vi "setup_lc_zt.vi"(0 "shuoming":string, 1 "didian":string, 6 "jsren":string, 9 "yw":string, 10 "id":string, 11 "zc_luodi_num":string) -> (2 "error":errorcluster caption="error out 2")   [LabVIEW 2017, in "Lib_code.lvlib"]
uses:
  Lib_code.lvlib
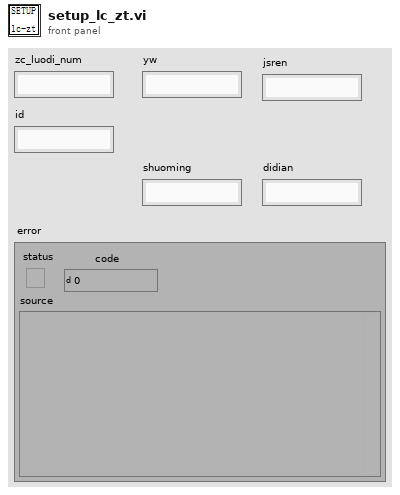
[diagram p1: front panel]
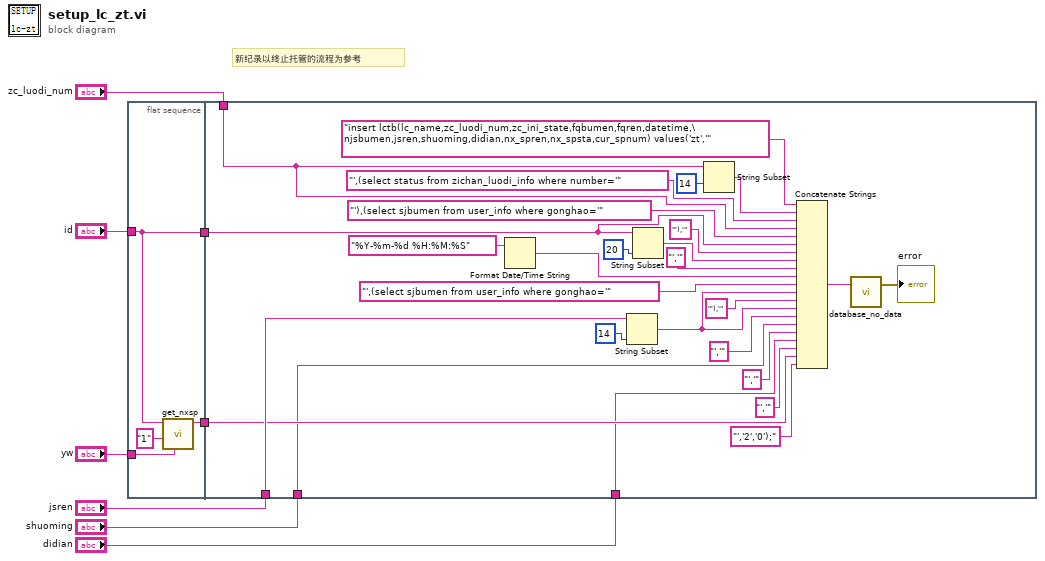
[diagram p0: block diagram]
diagram:
  # "新纪录以终止托管的流程为参考"
  n1 = flat-sequence {
    tunnel: "id" -> [w11]
    tunnel: [w11] -> w7
    tunnel: [w12] -> w6
    tunnel: "yw" -> [w10]
    tunnel: w7 -> [w20]
    tunnel: w6 -> [w28]
    tunnel: "zc_luodi_num" -> [w22]
    tunnel: "jsren" -> [w29]
    tunnel: "shuoming" -> [w16]
    tunnel: "didian" -> [w25]
    frame #0 {
      n2 = call "get_nxsp.vi"("yw"=w10, "Cur_state"="1", "fqren"=w11) -> ("sp_gonghao"=w12:string)  [unwired: 6 in, 2 out]
    }
    frame #1 {
      n3 = Format Date/Time String(time format string (%c)="%Y-%m-%d %H:%M:%S" ("时间格式字符串(%c)")) -> (date/time string=w15:string)  [unwired: 2 in]
      n4 = String Subset(string=w29, length (rest)=14 ("长度（剩余）")) -> (substring=w13:string)  [unwired: 1 in]
      n5 = String Subset(string=w20, length (rest)=20 ("长度（剩余）")) -> (substring=w32:string)  [unwired: 1 in]
      n6 = String Subset(string=w22, length (rest)=14 ("长度（剩余）")) -> (substring=w37:string)  [unwired: 1 in]
      n7 = Concatenate Strings("insert lctb(lc_name,zc_luodi_num,zc_ini_state,fqbumen,fqren,datetime,\njsbumen,jsren,shuoming,didian,nx_spren,nx_spsta,cur_spnum) values('zt','" ("格式字符串"), w37, "',(select status from zichan_luodi_info where number='" ("字符串"), w22, "'),(select sjbumen from user_info where gonghao='" ("字符串"), w20, "'),'" ("字符串"), w32, "','" ("字符串"), w15, "',(select sjbumen from user_info where gonghao='" ("字符串"), w13, "'),'" ("字符串"), w13, "','" ("字符串"), w16, "','" ("字符串"), w25, "','" ("字符串"), w28, "','2','0');" ("字符串")) -> (w27:string)
      n8 = call "database_no_data.vi"("input"=w27) -> ("error"=→"error":errorcluster)  [unwired: 2 in]
    }
  }
